vi "Initiate Data Log.vi"(8 "error in (no error)":errorcluster {"code" format="%.0x"}, 9 "Location (0: Internal)":i32(ring) items=["Internal", "External"], 10 "Data Log File Path (data1.dlog)":string="data1.dlog", 11 "VISA resource name":refnum<visa-resource-name>) -> (0 "error out":errorcluster {"code" format="%.0x"}, 3 "VISA resource name out":refnum<visa-resource-name>)   [LabVIEW 2016, in "Agilent N6700 Series.lvlib"]
doc: "Initiates the data logger. After you call this VI, the instrument leaves the idle state and waits for a trigger.\n\n<b>Note:</b>\nThis VI only applies to the N6705B and N6705C DC Power Analyzer."
uses:
  <instrlib>/Agilent N6700 Series/Agilent N6700 Series.lvlib
panel:
  # "The data log file path must include a .dlog file extension \nand can only be saved to an existing folder."
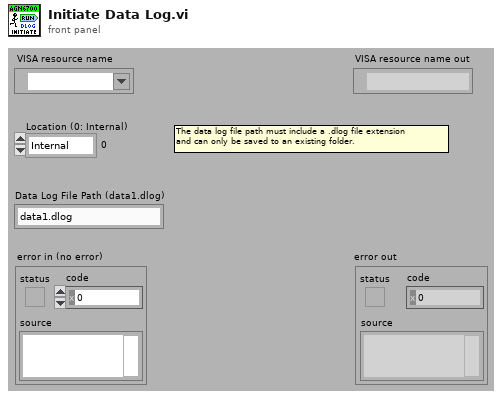
[diagram p1: front panel]
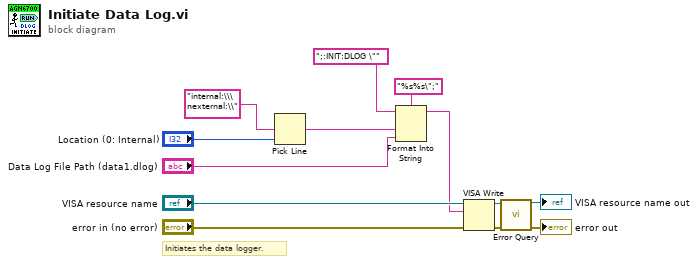
[diagram p0: block diagram]
diagram:
  # "Initiates the data logger."
  n1 = Pick Line(multi-line string="internal:\\\nexternal:\\", line index="Location (0: Internal)") -> (output string=w1:string)  [unwired: 1 in]
  n2 = Format Into String(format string="%s%s\";", initial string=";:INIT:DLOG \"" ("string"), w1, "Data Log File Path (data1.dlog)") -> (resulting string=w6:string)  [unwired: 1 in, 1 out]
  n3 = VISA Write(VISA resource name="VISA resource name", write buffer=w6, error in (no error)="error in (no error)") -> (VISA resource name out=w9:refnum<visa-resource-name>, error out=w8:errorcluster)  [unwired: 1 out]
  n4 = call <instrlib>:"Error Query.vi"("VISA resource name"=w9, "error in (no error)"=w8) -> ("VISA resource name out"=→"VISA resource name out":refnum<visa-resource-name>, "error out"=→"error out":errorcluster)  [unwired: 10 in, 2 out]
